vi "MovePIMotor.vi"(0 "System no.":i32=1 min=1 step=1, 5 "error in":errorcluster, 12 "Stop refnum":refnum<vi>) -> (19 "error out":errorcluster)   [LabVIEW 2013]
doc: "This VI is runs in a loop until the stop button is pressed, the stop reference is TRUE or an error occures. It lets the operator set the velocity, move the connected axes to relative, absolute or to the home position, and reads the current position continuosly. The diagram shows how to combine the driver and support VIs for these tasks. Use the Help?Show Context Help menu sequence in the LabVIEW environment to display the Context Help window with the VI and control/indicator descriptions.\nRun \" XXXX_Configuration_Setup.vi\" (with XXXX being the PI product number of your system) prior to running this VI. \n\nValid for: C-843, C-843.PM, C-865, C-866, Mercury"
uses:
  C:/Users/Public/PI/GCSMergedLabVIEW/Low Level/General command.llb/Global2 (Array).vi
panel:
  in  "Clear":bool
  in  "Define home":bool
  in  "Go home":bool
  in  "Move absolute":bool
  in  "Move relative (+)":bool
  in  "Move relative (-)":bool
  in  "Move":dbl[](array[numeric]) format="%.6f"
  out "Position":dbl[](array[numeric]) format="%.6f"
  in  "stop":bool
  out "Conn. Axes":string[](array[string])
  # "Command move:"
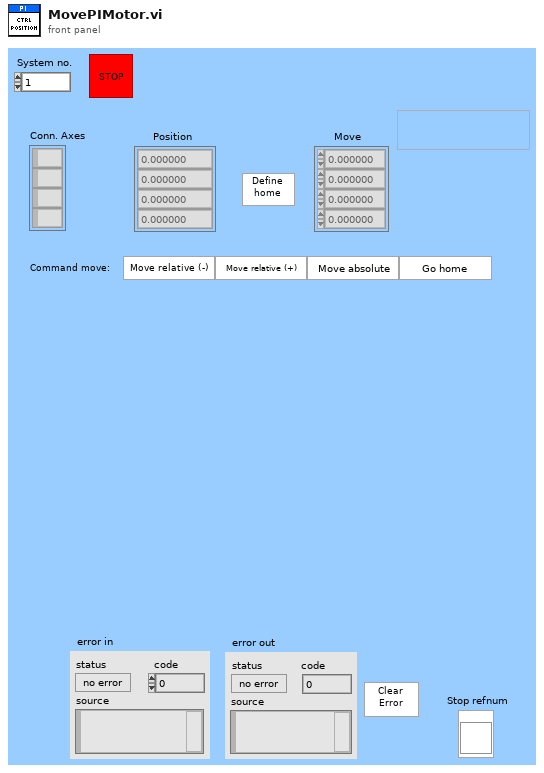
[diagram p1: front panel]
types:
  T1 = typedef "Controller names.ctl" = enum16{"None", "Analog", "C-702", "C-413", "C-843", "C-843.PM", "C-844", "C-848", "C-865", "C-866", "C-867", "C-877", "C-880", "C-884", "C-885", "C-891", "E-516", "E-517", "E-518", "E-709", "E-710", "E-712", "E-725", "E-727", "E-753", "E-754", "E-755", "E-761", "E-816", "E-861", "E-870", "E-871", "E-873", "F-206", "HydraPollux", "M-840", "M-850", "M-8X0", "Mercury", "Mercury_GCS"}
  T2 = cluster{"Conn. axes":string[], "Controller name":T1}[]
  T3 = cluster{"Conn. axes":string[], "Controller name":T1}
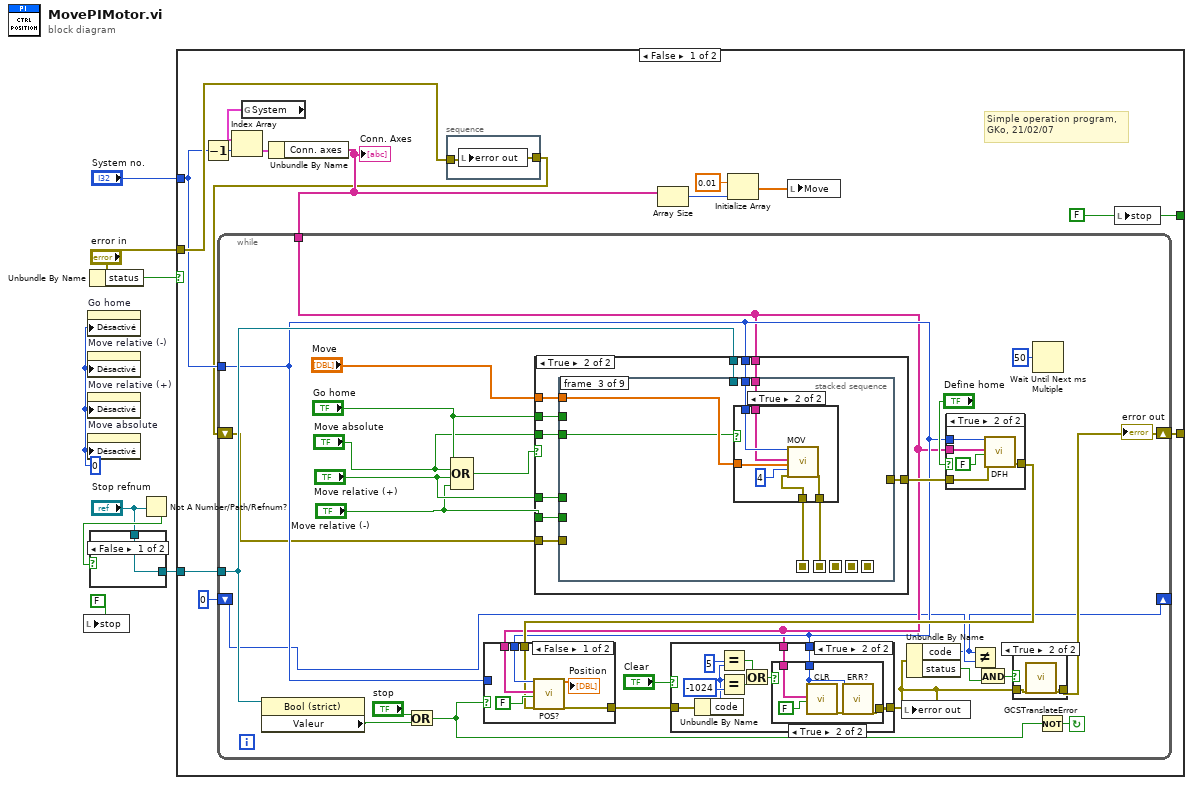
[diagram p0: block diagram]
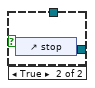
[diagram p2: hidden frame]
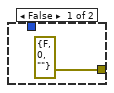
[diagram p5: hidden frame]
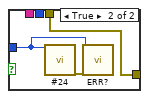
[diagram p6: hidden frame]
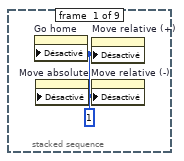
[diagram p8: hidden frame]
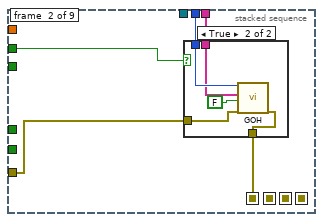
[diagram p9: hidden frame]
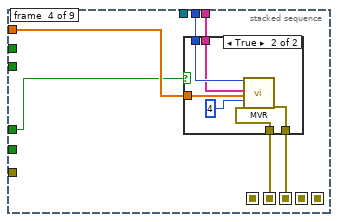
[diagram p12: hidden frame]
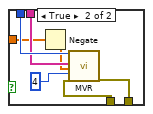
[diagram p15: hidden frame]
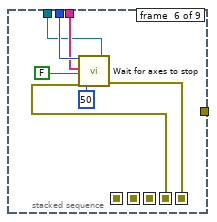
[diagram p16: hidden frame]
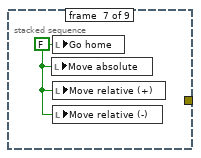
[diagram p17: hidden frame]
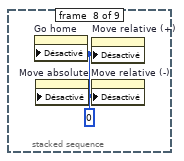
[diagram p18: hidden frame]
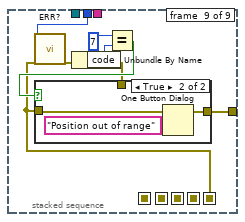
[diagram p19: hidden frame]
diagram:
  w2 = u8 0 ("Disabled")
  # "Simple operation program,\nGKo, 21/02/07"
  n1 = local write "stop"(FALSE ("stop")) -> ()
  n2 = property on="Go home" class="Bool (strict)"("Désactivé"=w2) -> ()  [unwired: 2 in, 2 out]
  n3 = property on="Move relative (-)" class="Bool (strict)"("Désactivé"=w2) -> ()  [unwired: 2 in, 2 out]
  n4 = property on="Move relative (+)" class="Bool (strict)"("Désactivé"=w2) -> ()  [unwired: 2 in, 2 out]
  n5 = property on="Move absolute" class="Bool (strict)"("Désactivé"=w2) -> ()  [unwired: 2 in, 2 out]
  n6 = Unbundle By Name("error in") -> ("status"=w9:bool)
  n7 = Not A Number/Path/Refnum?(number/path/refnum="Stop refnum") -> (NaN/Path/Refnum?=w6:bool)
  n8 = case shown="False" w6 {
    tunnel: [w11 w12] -> w5
    tunnel: "Stop refnum" -> [w11 _]
    frame False {
    }
    frame True {
      n9 = control-ref of="stop"() -> (w12:refnum<vi>)
    }
  }
  n10 = case shown="False" w9 {
    tunnel: [w26 w173] -> w8
    tunnel: "error in" -> [w25 w173]
    tunnel: "System no." -> [w18 _]
    tunnel: w5 -> [w24 _]
    tunnel: [FALSE ("stop") FALSE ("stop")] -> w1
    frame False {
      n11 = Decrement(x=w18) -> (x-1=w17:i32)
      n12 = global read "Global2 (Array).vi" "System"() -> (w16:T2)
      n13 = Index Array(array=w16, index=w17) -> (element=w15:T3)
      n14 = Unbundle By Name(w15) -> ("Conn. axes"=w14:string[])
      "Conn. Axes" <- w14
      n15 = stacked-sequence {
        tunnel: w25 -> [w171]
        tunnel: [w171] -> w13
        frame #0 {
          n16 = local write "error out"(w171) -> ()
        }
      }
      n17 = while {
        shift-left: 0 ("code") -> [w37]
        shift-right: [w36] -> _
        tunnel: w24 -> [w46]
        tunnel: w14 -> [w38]
        shift-left: w13 -> [w28]
        shift-right: [w40] -> w26
        tunnel: w18 -> [w39]
        stop <- w53 continue-if-true
        n18 = property class="Bool (strict)"(reference=w46) -> ("Valeur"=w47:bool)  [unwired: 1 in, 2 out]
        n19 = Or(x="stop", y=w47) -> (x .or. y?=w41:bool)
        n20 = Compound Arithmetic op=OR("Go home", "Move absolute", "Move relative (+)", "Move relative (-)") -> (w27:bool)
        n21 = case shown="True" w27 {
          tunnel: "Go home" -> [_ w93]
          tunnel: w39 -> [_ w92]
          tunnel: w38 -> [_ w91]
          tunnel: "Move" -> [_ w90]
          tunnel: [w83 w89] -> w45
          tunnel: "Move relative (-)" -> [_ w88]
          tunnel: w46 -> [_ w87]
          tunnel: "Move absolute" -> [_ w86]
          tunnel: "Move relative (+)" -> [_ w85]
          tunnel: w28 -> [w83 w84]
          frame False {
          }
          frame True {
            n22 = stacked-sequence {
              seq-local: [_ w96 _ _ _ _ _ _ _] -> [_ _ w109 _ _ _ _ _ _]
              seq-local: [_ _ w107 _ _ _ _ _ _] -> [_ _ _ w120 _ _ _ _ _]
              seq-local: [_ _ _ w121 _ _ _ _ _] -> [_ _ _ _ w133 _ _ _ _]
              seq-local: [_ _ _ _ w132 _ _ _ _] -> [_ _ _ _ _ w152 _ _ _]
              seq-local: [_ _ _ _ _ w146 _ _ _] -> [_ _ _ _ _ _ _ _ w155]
              tunnel: w93 -> [_ w99 _ _ _ _ _ _ _]
              tunnel: w92 -> [_ w98 w111 w124 w137 w151 _ _ w161]
              tunnel: w91 -> [_ w97 w110 w123 w136 w150 _ _ _]
              tunnel: w90 -> [_ _ w108 w122 w135 _ _ _ _]
              tunnel: [_ _ _ _ _ _ _ _ w157] -> w89
              tunnel: w88 -> [_ _ _ _ w134 _ _ _ _]
              tunnel: w87 -> [_ _ _ _ _ w147 _ _ _]
              tunnel: w86 -> [_ _ w106 _ _ _ _ _ _]
              tunnel: w85 -> [_ _ _ w119 _ _ _ _ _]
              tunnel: w84 -> [_ w95 _ _ _ _ _ _ _]
              frame #0 {
                w94 = u8 1 ("Disabled")
                n23 = property on="Go home" class="Bool (strict)"("Désactivé"=w94) -> ()  [unwired: 2 in, 2 out]
                n24 = property on="Move absolute" class="Bool (strict)"("Désactivé"=w94) -> ()  [unwired: 2 in, 2 out]
                n25 = property on="Move relative (+)" class="Bool (strict)"("Désactivé"=w94) -> ()  [unwired: 2 in, 2 out]
                n26 = property on="Move relative (-)" class="Bool (strict)"("Désactivé"=w94) -> ()  [unwired: 2 in, 2 out]
              }
              frame #1 {
                n27 = case shown="True" w99 {
                  tunnel: w98 -> [_ w105]
                  tunnel: w97 -> [_ w104]
                  tunnel: [w100 w102] -> w96
                  tunnel: w95 -> [w100 w101]
                  frame False {
                  }
                  frame True {
                    n28 = call "GOH.vi"("System no."=w105, "GOH axes"=w104, "All axes?"=FALSE, "error in"=w101) -> ("error out"=w102:errorcluster)  [unwired: 15 in]
                  }
                }
              }
              frame #2 {
                n29 = case shown="True" w106 {
                  tunnel: w111 -> [_ w118]
                  tunnel: w110 -> [_ w117]
                  tunnel: w109 -> [w112 w115]
                  tunnel: w108 -> [_ w114]
                  tunnel: [w112 w113] -> w107
                  frame False {
                  }
                  frame True {
                    n30 = call "MOV.vi"("System no."=w118, "Axes to move"=w117, "Position values"=w114, "No.of digits"=i16 4, "error in"=w115) -> ("error out"=w113:errorcluster)  [unwired: 14 in]
                  }
                }
              }
              frame #3 {
                n31 = case shown="True" w119 {
                  tunnel: w124 -> [_ w131]
                  tunnel: w123 -> [_ w130]
                  tunnel: w122 -> [_ w129]
                  tunnel: [w125 w127] -> w121
                  tunnel: w120 -> [w125 w126]
                  frame False {
                  }
                  frame True {
                    n32 = call "MVR.vi"("System no."=w131, "Axes to move"=w130, "Position values"=w129, "No.of digits"=i16 4, "error in"=w126) -> ("error out"=w127:errorcluster)  [unwired: 14 in]
                  }
                }
              }
              frame #4 {
                n33 = case shown="False" w134 {
                  tunnel: w137 -> [_ w145]
                  tunnel: w136 -> [_ w144]
                  tunnel: w135 -> [_ w142]
                  tunnel: w133 -> [w138 w140]
                  tunnel: [w138 w139] -> w132
                  frame False {
                  }
                  frame True {
                    n34 = Negate(x=w142) -> (-x=w141:dbl[])
                    n35 = call "MVR.vi"("System no."=w145, "Axes to move"=w144, "Position values"=w141, "No.of digits"=i16 4, "error in"=w140) -> ("error out"=w139:errorcluster)  [unwired: 14 in]
                  }
                }
              }
              frame #5 {
                n36 = call "Wait for axes to stop.vi"("System no."=w151, "Axes to wait for"=w150, "With status bit polling?"=FALSE, "error in"=w152, "Polling cycle time, ms"=u32 50, "Stop refnum"=w147) -> ("error out"=w146:errorcluster)  [unwired: 12 in, 1 out]
              }
              frame #6 {
                w153 = FALSE ("Go home")
                n37 = local write "Move absolute"(w153) -> ()
                n38 = local write "Go home"(w153) -> ()
                n39 = local write "Move relative (+)"(w153) -> ()
                n40 = local write "Move relative (-)"(w153) -> ()
              }
              frame #7 {
                w154 = u8 0 ("Disabled")
                n41 = property on="Go home" class="Bool (strict)"("Désactivé"=w154) -> ()  [unwired: 2 in, 2 out]
                n42 = property on="Move absolute" class="Bool (strict)"("Désactivé"=w154) -> ()  [unwired: 2 in, 2 out]
                n43 = property on="Move relative (+)" class="Bool (strict)"("Désactivé"=w154) -> ()  [unwired: 2 in, 2 out]
                n44 = property on="Move relative (-)" class="Bool (strict)"("Désactivé"=w154) -> ()  [unwired: 2 in, 2 out]
              }
              frame #8 {
                n45 = call "ERR?.vi"("System no."=w161, "error in"=w155) -> ("error out"=w156:errorcluster)  [unwired: 16 in, 1 out]
                n46 = Unbundle By Name(w156) -> ("code"=w159:i32)
                n47 = Equal?(x=7 ("y"), y=w159) -> (x = y?=w158:bool)
                n48 = case shown="True" w158 {
                  tunnel: [w162 w163] -> w157
                  tunnel: w156 -> [w162 _]
                  tunnel: w155 -> [_ w163]
                  frame False {
                  }
                  frame True {
                    n49 = One Button Dialog(message="Position out of range") -> ()  [unwired: 1 in, 1 out]
                  }
                }
              }
            }
          }
        }
        n50 = case shown="True" "Define home" {
          tunnel: w39 -> [_ w170]
          tunnel: w38 -> [_ w169]
          tunnel: w45 -> [w165 w167]
          tunnel: [w165 w166] -> w44
          frame False {
          }
          frame True {
            n51 = call "DFH.vi"("System no."=w170, "DFH axes"=w169, "All axes?"=FALSE, "error in"=w167) -> ("error out"=w166:errorcluster)  [unwired: 15 in]
          }
        }
        n52 = case shown="False" w41 {
          tunnel: w39 -> [_ w81]
          tunnel: w38 -> [w77 _]
          tunnel: w39 -> [w76 _]
          tunnel: w44 -> [w75 w80]
          tunnel: [w74 w80] -> w42
          frame False {
            n53 = call "POS?.vi"("System no."=w76, "Axes to query"=w77, "All axes?"=FALSE, "error in"=w75) -> ("Position"=→"Position":dbl[], "error out"=w74:errorcluster)  [unwired: 14 in]
          }
          frame True {
            n54 = call "#24.vi"("System no."=w81) -> ("error out"=w82:errorcluster)  [unwired: 18 in]
            n55 = call "ERR?.vi"("System no."=w81, "error in"=w82) -> ()  [unwired: 16 in, 2 out]
          }
        }
        n56 = case shown="True" "Clear" {
          tunnel: [w57 w60] -> w33
          tunnel: w42 -> [w57 w64]
          tunnel: w39 -> [_ w59]
          tunnel: w38 -> [_ w58]
          frame False {
          }
          frame True {
            n57 = Unbundle By Name(w64) -> ("code"=w65:i32)
            n58 = Equal?(x=5 ("y"), y=w65) -> (x = y?=w63:bool)
            n59 = Equal?(x=w65, y=-1024) -> (x = y?=w61:bool)
            n60 = Or(x=w63, y=w61) -> (x .or. y?=w62:bool)
            n61 = case shown="True" w62 {
              tunnel: [errorcluster {"status"=FALSE, "code"=0, "source"=""} ("error out") w72] -> w60
              tunnel: w59 -> [_ w71]
              tunnel: w58 -> [_ w70]
              frame False {
              }
              frame True {
                n62 = call "CLR.vi"("System no."=w71, "CLR axes"=w70, "All axes?"=FALSE) -> ("error out"=w73:errorcluster)  [unwired: 16 in]
                n63 = call "ERR?.vi"("System no."=w71, "error in"=w73) -> ("error out"=w72:errorcluster)  [unwired: 16 in, 1 out]
              }
            }
          }
        }
        n64 = local write "error out"(w33) -> ()
        n65 = Unbundle By Name(w33) -> ("code"=w36:i32, "status"=w32:bool)
        n66 = Not Equal?(x=w36, y=w37) -> (x != y?=w35:bool)
        n67 = And(x=w35, y=w32) -> (x .and. y?=w34:bool)
        n68 = case shown="True" w34 {
          tunnel: w33 -> [w54 w56]
          tunnel: [w54 w55] -> w40
          frame False {
          }
          frame True {
            n69 = call "GCSTranslateError.vi"("error in"=w56) -> ("error out"=w55:errorcluster)  [unwired: 16 in, 2 out]
          }
        }
        n70 = Wait Until Next ms Multiple(millisecond multiple=u32 50) -> ()  [unwired: 1 out]
        n71 = Not(x=w41) -> (.not. x?=w53:bool)
      }
      n72 = Array Size(array=w14) -> (size(s)=w22:i32)
      n73 = Initialize Array(0.01 ("Move"), w22) -> (w21:dbl[])
      n74 = local write "Move"(w21) -> ()
    }
    frame True {
    }
  }
  "error out" <- w8
  n75 = local write "stop"(w1) -> ()
